vi "Flatten and Get String Property.vi"(8 "error in (no error)":errorcluster, 9 "Default Value":variant, 10 "Property Name":string, 11 "Section Ref in":T1 format="%.0x") -> (0 "error out":errorcluster, 1 "Value":variant, 3 "Section Ref out":T1 format="%.0x")   [LabVIEW 2015, in "NI 9759 RevB Custom Device.lvlib"]
uses:
  NI 9759 RevB Custom Device.lvlib
  <vilib>/NI Veristand/Custom Device API/Custom Device Item Ref.ctl
  <vilib>/NI Veristand/Custom Device API/Get Item Property (String).vi
  <vilib>/NI VeriStand/Custom Device API/Custom Device API.lvlib
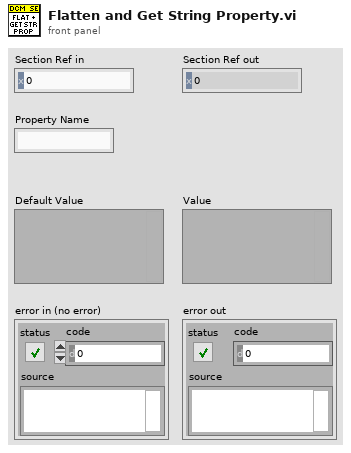
[diagram p1: front panel]
types:
  T1 = typedef "Custom Device API.lvlib/Custom Device Item Ref.ctl" = u64
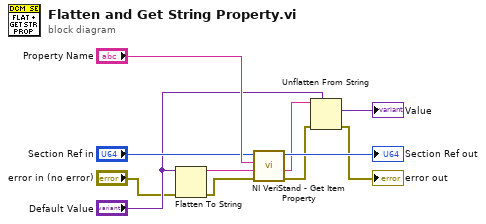
[diagram p0: block diagram]
diagram:
  n1 = Flatten To String(anything="Default Value", error in (no error)="error in (no error)") -> (data string=w7:string, error out=w3:errorcluster)  [unwired: 2 in, 1 out]
  n2 = call-poly <vilib>:"NI VeriStand - Get Item Property.vi"("error in (no error)"=w3, "Default Value"=w7, "Property Name"="Property Name", "Item Ref in"="Section Ref in") -> ("error out"=w2:errorcluster, "Value"=w8:string, "Item Ref out"=→"Section Ref out":T1)  [unwired: 4 in, 1 out]
  n3 = Unflatten From String(type="Default Value", binary string=w8, error in (no error)=w2) -> (value=→"Value":variant, error out=→"error out":errorcluster)  [unwired: 2 in, 1 out]
